vi "Before Write.vi"(6 "State In":variant, 7 "Compiled Inline Async Settings":variant, 8 "error in":errorcluster, 9 "Custom Settings":variant, 10 "Compiled Settings":variant, 11 "Custom Device API in":refnum<class "Custom Device API.lvclass">) -> (0 "error out":errorcluster, 3 "Custom Device API out":refnum<class "Custom Device API.lvclass">, 4 "State Out":variant)   [LabVIEW 2026, in "Template Debug Tools.lvlib"]
uses:
  Template Debug Tools.lvlib
  <userlib>/Custom Device Interfaces_v1.lvlibp/CustomDeviceAPI/Custom Device API.lvclass
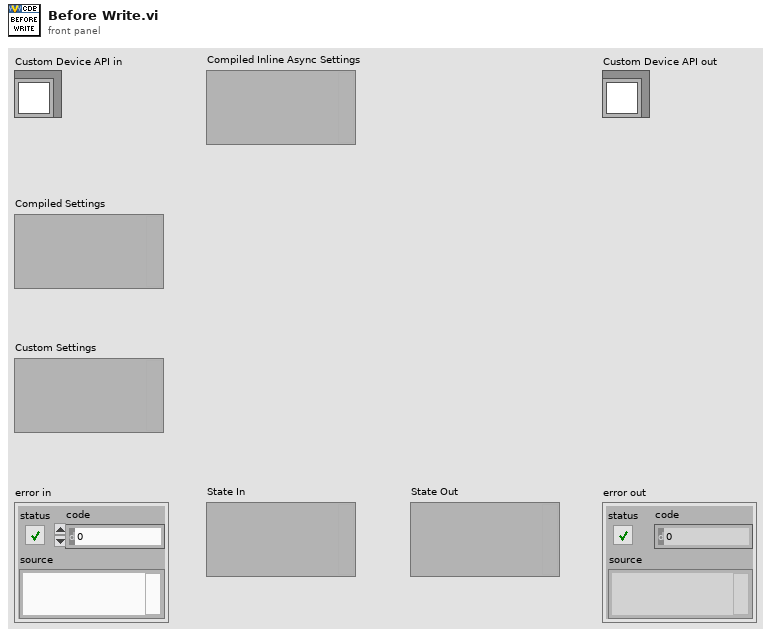
[diagram p1: front panel]
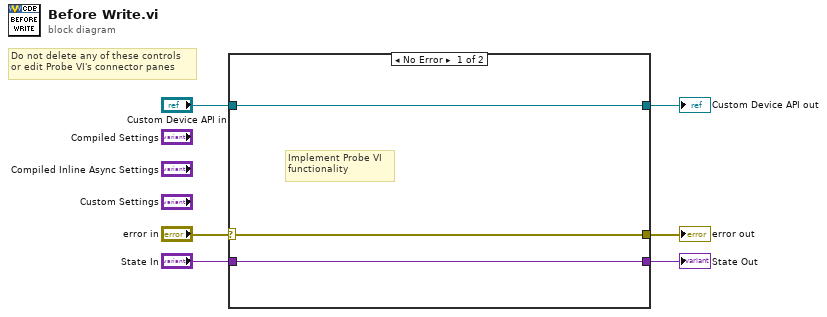
[diagram p0: block diagram]
diagram:
  # "Do not delete any of these controls\nor edit Probe VI's connector panes"
  n1 = case shown="No Error" "error in" {
    selector: "error in" -> [w9 w11]
    tunnel: [w9 w11] -> w5
    tunnel: "Custom Device API in" -> [w8 w12]
    tunnel: [w8 w12] -> w3
    tunnel: "State In" -> [w7 w10]
    tunnel: [w7 w10] -> w1
    frame No Error {
      # "Implement Probe VI\nfunctionality"
    }
    frame Error {
    }
  }
  "Custom Device API out" <- w3
  "error out" <- w5
  "State Out" <- w1
